vi "Event handler-Update AOL globals on UI events.vi"(8 "error in (no error)":errorcluster) -> (0 "error out":errorcluster)   [LabVIEW 2020]
uses:
  Global Variables/gl_UI Ctrl Refs.vi
  Global Variables/General Globals.vi
  Configuration code/Calibration/Globals/gl_Calibration globals.vi
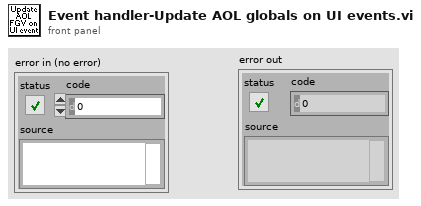
[diagram p1: front panel]
types:
  T1 = typedef "UI ctrl refs cluster.ctl" = cluster{"Top level VI path":path, "Top level VI ref":refnum<vi>, "User menu ref":refnum<k9>, "Sub Panel control":refnum<vi>, "Imaging Param Tab":refnum<vi>, "Occurrence-Start drivers":refnum<k4>, "Occurrence-Speed logging initialised":refnum<k4>, "Occurrence-XYZ stage initialised":refnum<k4>, "Exit button":refnum<vi>, "Status ind":refnum<vi>, "Set as origin":refnum<vi>, "Speed Logging":refnum<vi>, "Time Lapse":refnum<vi>, "Live Imaging":refnum<vi>, "AOL Z Stack":refnum<vi>, "Motor Z Stack":refnum<vi>, "Funct Acq button":refnum<vi>, "Hard Shutter":refnum<vi>, "Virtual Shutter":refnum<vi>, "Laser Power":refnum<vi>, "AOL Mode":refnum<vi>, "Frame Size":refnum<vi>, "Field of View":refnum<vi>, "Dwell Time":refnum<vi>, "Zoom":refnum<vi>, "AOL Z":refnum<vi>, "Objective":refnum<vi>, "Axis":refnum<vi>, "Paths & Names":refnum<vi>, "Experiment folder path (ind.)":refnum<vi>, "Last State (Ind.)":refnum<vi>, "Averages":refnum<vi>, "Angle (degrees)":refnum<vi>, "X centre":refnum<vi>, "Y centre":refnum<vi>, "Plane Mode":refnum<vi>, "# Planes":refnum<vi>, "Z Start":refnum<vi>, "Z Stop":refnum<vi>, "Z Step":refnum<vi>, "PMT 1":refnum<vi>, "PMT 2":refnum<vi>, "Stage XYZ Position":refnum<vi>, "Pockels@Z Start":refnum<vi>, "Pockels@Z Stop":refnum<vi>, "Obtain Z Start":refnum<vi>, "Obtain Z Stop":refnum<vi>, "Live stim.trig.period":refnum<vi>, "Live stim.trig.enable":refnum<vi>, "Movement Correction":refnum<vi>, "Load Reference Image":refnum<vi>, "XY Stage Move":refnum<vi>, "MovCor Cluster":refnum<vi>, "RefDAQParam":refnum<vi>, "Funct. Acq. Pockels Modulation":refnum<vi>, "Ref Laser Power":refnum<vi>, "Enable Video Recording":refnum<vi>, "Video Record-Live Imaging":refnum<vi>, "Video Record-Funct acq":refnum<vi>, "Reference Source":refnum<vi>, "AOL Z-stack Chirps Ready (ind)":refnum<vi>, "Target time between mov.cor. ref triggers (ms)":refnum<vi>, "Funct. Acq. Ref frame save":refnum<vi>, "Tracking button":refnum<vi>, "Show ref plots window":refnum<vi>, "Center freq ind (nm)":refnum<vi>, "Pickup mode (ind)":refnum<vi>, "Logging queue (ind)":refnum<vi>, "Back aperture power (ind.)":refnum<vi>, "Power after objective (ind.)":refnum<vi>, "Switch user":refnum<vi>, "Ls1 Conn. Status":refnum<vi>, "Ls1Tuning Status":refnum<vi>, "Ls1 Faults":refnum<vi>, "Ls1 Connection":refnum<vi>, "Ls1 Mode":refnum<vi>, "Ls1 POWER [mW]":refnum<vi>, "Ls1Shutter":refnum<vi>, "Ls1 Wavelength":refnum<vi>, "Ls1 Note":refnum<vi>, "Ls1 Confirm Wav":refnum<vi>, "Ls1 PreChrp Prism1":refnum<vi>, "Ls1 PreChrp Prism2":refnum<vi>, "Ls1 wav top Ind":refnum<vi>, "Ls1 power top Ind":refnum<vi>, "Ls1 Pump peak Hold":refnum<vi>, "Ls1 Status Ind":refnum<vi>, "Ls1 wav cancel":refnum<vi>, "Experiment Type":refnum<vi>, "Biology Information":refnum<vi>, "Camera recording status":refnum<vi>}
  T2 = typedef "AOL_Globals.ctl" = cluster{"Imaging Protocol":T3, "Number of POI":u16, "Number of Miniscans":u16, "Number of Trials":u16, "Number of Cycles ":u64, "# Averaged Frames":u16, "Laser power (%)":u8, "Pockels (V)":dbl, "Acquisition Length (sec)":dbl, "Fill time (us)":dbl, "POI Dwell time (us)":dbl, "Miniscan Dwell time per pixel (us)":dbl, "PMT 1":dbl, "PMT 2":dbl, "Back Apperture (mA)":dbl, "Frame Size":T4, "Center Frequency":dbl, "Field of View (norm)":dbl, "DwellTime (us)":dbl, "Wavelength (nm)":dbl, "Zoom":dbl, "AOL Z":dbl, "AOL Mode":T5, "GridXY":dbl, "GridZ":dbl, "TriggerPeriod (sec)":dbl, "Number of Pixels in Miniscan":u16, "Experiment folder path":path, "X centre":dbl, "Y centre":dbl, "Angle (degrees)":dbl, "Plane Mode":T6, "Threshold":u16[], "Regenerate Chirps":bool, "Rectangle ROI length (pixels)":u16, "Rectangle ROI height (pixels)":u16, "AOD fill":u16, "StartupDelay":i32, "Samples Wait after Trigger":u16, "Slip Cycle":u32, "Add Cycle":bool, "Functional Mode":T7, "Z Start":dbl, "Z Stop":dbl, "# Planes":i32, "Total Pixels":i32, "Variable Miniscan Pixels":u16[], "Use Variable Length":bool, "Use Variable Resolution":bool, "Laser power (%) at Z Start":u8, "Laser power (%) at Z Stop":u8, "Ref Z Step":i8, "Ref Dwell Time (us)":dbl, "Field of View (um)":dbl}
  T3 = typedef "Imaging Protocols enum.ctl" = enum16{"AOL Z-Stack", "Motor Z Stack", "Functional Acquisition", "Single Plane Acquisition", "Volume Acquisition", "Live Imaging", "Live Plane Imaging", "Live Volume Imaging"}
  T4 = typedef "Frame Size.ctl" = u16
  T5 = typedef "AOL modes.ctl" = enum16{"Raster", "Structural", "Pointing", "Mini Scan", "Alignment"}
  T6 = typedef "Plane Mode.ctl" = u16
  T7 = typedef "Functional Mode.ctl" = enum16{"Point", "Line", "Patch", "Plane", "Volume"}
  T8 = typedef "Laser control knob.ctl" = u16
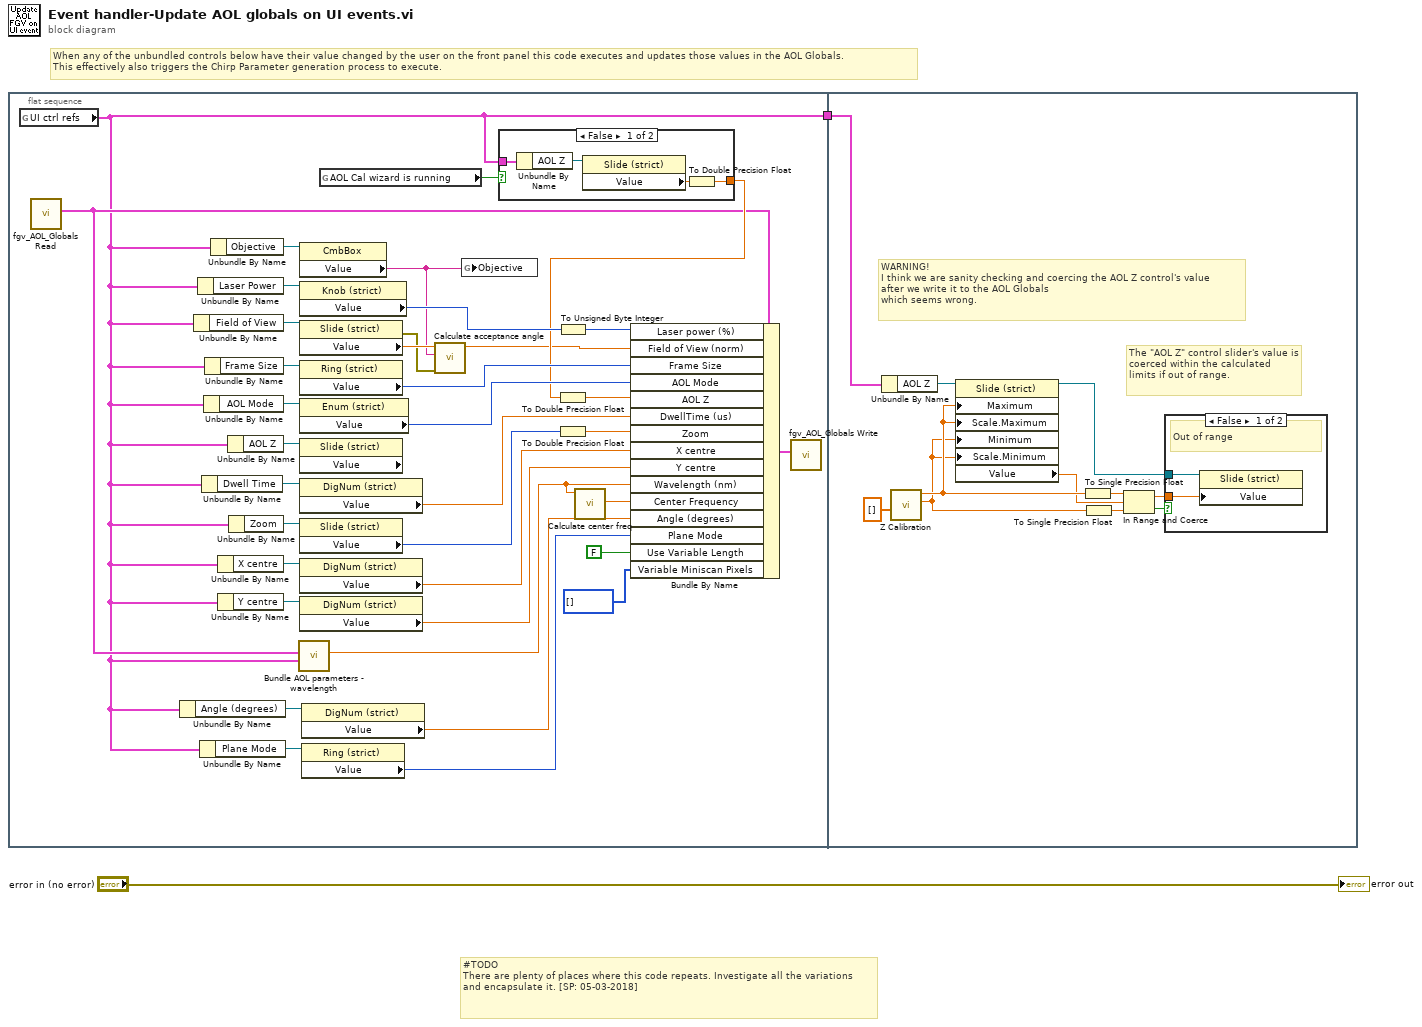
[diagram p0: block diagram]
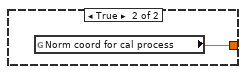
[diagram p2: hidden frame]
diagram:
  # "#TODO\nThere are plenty of places where this code repeats. Investigate all the variations\nand encapsulate it. [SP: 05-03-2018]"
  # "When any of the unbundled controls below have their value changed by the user on the front panel this code executes and updates those values in the AOL Globals.\nThis effectively also triggers the Chirp Parameter generation process to execute."
  n1 = flat-sequence {
    tunnel: [w6] -> w2
    tunnel: w2 -> [w48]
    frame #0 {
      n2 = global read "gl_UI Ctrl Refs.vi" "UI ctrl refs"() -> (w6:T1)
      n3 = call "fgv_AOL_Globals Read.vi"() -> ("AOL_Globals"=w7:T2)  [unwired: 9 in, 2 out]
      n4 = Unbundle By Name(w6) -> ("Angle (degrees)"=w24:refnum<vi>)
      n5 = Unbundle By Name(w6) -> ("Field of View"=w37:refnum<vi>)
      n6 = Unbundle By Name(w6) -> ("Laser Power"=w38:refnum<vi>)
      n7 = Unbundle By Name(w6) -> ("Plane Mode"=w25:refnum<vi>)
      n8 = Unbundle By Name(w6) -> ("Dwell Time"=w33:refnum<vi>)
      n9 = Unbundle By Name(w6) -> ("AOL Mode"=w35:refnum<vi>)
      n10 = Unbundle By Name(w6) -> ("Frame Size"=w36:refnum<vi>)
      n11 = Unbundle By Name(w6) -> ("Objective"=w27:refnum<vi>)
      n12 = Unbundle By Name(w6) -> ("X centre"=w22:refnum<vi>)
      n13 = Unbundle By Name(w6) -> ("Y centre"=w23:refnum<vi>)
      n14 = Unbundle By Name(w6) -> ("AOL Z"=w34:refnum<vi>)
      n15 = Unbundle By Name(w6) -> ("Zoom"=w32:refnum<vi>)
      n16 = call "Bundle AOL parameters - wavelength.vi"("UI ctrl refs"=w6, "AOL_Globals in"=w7) -> ("Wavelength"=w5:dbl)  [unwired: 9 in]
      n17 = property class="CmbBox"(reference=w27) -> ("Value"=w10:string)  [unwired: 1 in, 2 out]
      n18 = property class="Knob (strict)"(reference=w38) -> ("Value"=w31:T8)  [unwired: 1 in, 2 out]
      n19 = property class="Slide (strict)"(reference=w37) -> (error out=w8:errorcluster, "Value"=w11:sgl)  [unwired: 1 in, 1 out]
      n20 = property class="Ring (strict)"(reference=w36) -> ("Value"=w15:u16)  [unwired: 1 in, 2 out]
      n21 = property class="Enum (strict)"(reference=w35) -> ("Value"=w30:T5)  [unwired: 1 in, 2 out]
      n22 = property class="Slide (strict)" props=["Value"](reference=w34) -> ()  [unwired: 1 in, 3 out]
      n23 = property class="DigNum (strict)"(reference=w33) -> ("Value"=w29:dbl)  [unwired: 1 in, 2 out]
      n24 = property class="Slide (strict)"(reference=w32) -> ("Value"=w28:i8)  [unwired: 1 in, 2 out]
      n25 = property class="DigNum (strict)"(reference=w22) -> ("Value"=w21:dbl)  [unwired: 1 in, 2 out]
      n26 = property class="DigNum (strict)"(reference=w23) -> ("Value"=w20:dbl)  [unwired: 1 in, 2 out]
      n27 = property class="DigNum (strict)"(reference=w24) -> ("Value"=w19:dbl)  [unwired: 1 in, 2 out]
      n28 = property class="Ring (strict)"(reference=w25) -> ("Value"=w18:T6)  [unwired: 1 in, 2 out]
      n29 = global read "gl_Calibration globals.vi" "AOL Cal wizard is running"() -> (w14:bool)
      n30 = call "Calculate acceptance angle.vi"("error in (no error)"=w8, "Objective"=w10, "FOV (true)"=w11) -> ("Acceptance Angle (mrad)"=w9:dbl)  [unwired: 7 in, 1 out]
      n31 = global write "General Globals.vi" "Objective"(w10) -> ()
      n32 = case shown="False" w14 {
        tunnel: [w41 w44] -> w13
        tunnel: w6 -> [w40 _]
        frame False {
          n33 = Unbundle By Name(w40) -> ("AOL Z"=w43:refnum<vi>)
          n34 = property class="Slide (strict)"(reference=w43) -> ("Value"=w42:sgl)  [unwired: 1 in, 2 out]
          n35 = To Double Precision Float(number=w42) -> (double precision float=w41:dbl)
        }
        frame True {
          n36 = global read "gl_Calibration globals.vi" "Norm coord for cal process"() -> (w44:dbl)
        }
      }
      n37 = To Unsigned Byte Integer(number=w31) -> (unsigned 8bit integer=w16:u8)
      n38 = To Double Precision Float(number=w13) -> (double precision float=w17:dbl)
      n39 = To Double Precision Float(number=w28) -> (double precision float=w26:dbl)
      n40 = call "Calculate center freq.vi"("UI Wavelength"=w5) -> ("Centre frequency (MHz)"=w12:dbl)  [unwired: 9 in, 1 out]
      n41 = Bundle By Name(cluster=w7, "Laser power (%)"=w16, "Field of View (norm)"=w9, "Frame Size"=w15, "AOL Mode"=w30, "AOL Z"=w17, "DwellTime (us)"=w29, "Zoom"=w26, "X centre"=w21, "Y centre"=w20, "Wavelength (nm)"=w5, "Center Frequency"=w12, "Angle (degrees)"=w19, "Plane Mode"=w18, "Use Variable Length"=FALSE, "Variable Miniscan Pixels"=u16[] []) -> (w39:T2)
      n42 = call "fgv_AOL_Globals Write.vi"("AOL_Globals"=w39) -> ()  [unwired: 10 in, 1 out]
    }
    frame #1 {
      # "WARNING!\nI think we are sanity checking and coercing the AOL Z control's value\nafter we write it to the AOL Globals\nwhich seems wrong."
      # "The \"AOL Z\" control slider's value is coerced within the calculated limits if out of range."
      n43 = Unbundle By Name(w48) -> ("AOL Z"=w47:refnum<vi>)
      n44 = call "Z Calibration.vi"("Z Planes"=dbl[] [] ("Motor Z")) -> ("Z Min"=w46:dbl, "Z Max"=w54:dbl)  [unwired: 7 in, 2 out]
      n45 = property on="Property Node" class="Slide (strict)"(reference=w47, "Maximum"=w54, "Scale.Maximum"=w54, "Minimum"=w46, "Scale.Minimum"=w46) -> (reference out=w45:refnum<vi>, "Value"=w53:sgl)  [unwired: 1 in, 1 out]
      n46 = To Single Precision Float(number=w54) -> (single precision float=w52:sgl)
      n47 = To Single Precision Float(number=w46) -> (single precision float=w51:sgl)
      n48 = In Range and Coerce(upper limit=w52, x=w53, lower limit=w51) -> (coerced(x)=w49:sgl, In Range?=w50:bool)
      n49 = case shown="False" w50 {
        tunnel: w49 -> [w57 _]
        tunnel: w45 -> [w56 _]
        frame False {
          # "Out of range"
          n50 = property on="Property Node" class="Slide (strict)"(reference=w56, "Value"=w57) -> ()  [unwired: 1 in, 2 out]
        }
        frame True {
          # "In range"
        }
      }
    }
  }
  "error out" <- "error in (no error)"
